vi "Write perform dynamic reads.vi"(8 "error in":errorcluster, 10 "perform dynamic reads":bool, 11 "DecideProjectFeatures in":refnum<class "TagBusProcessingPluginFeatureDecider.lvclass">) -> (0 "error out":errorcluster, 3 "DecideProjectFeatures out":refnum<class "TagBusProcessingPluginFeatureDecider.lvclass">)   [LabVIEW 2013, in "TagBusProcessingPluginFeatureDecider.lvclass"]
uses:
  TagBusProcessingPluginFeatureDecider.lvclass
  TagBusProcessingPluginFeatureDecider.lvclass/TagBusProcessingPluginFeatureDecider.ctl
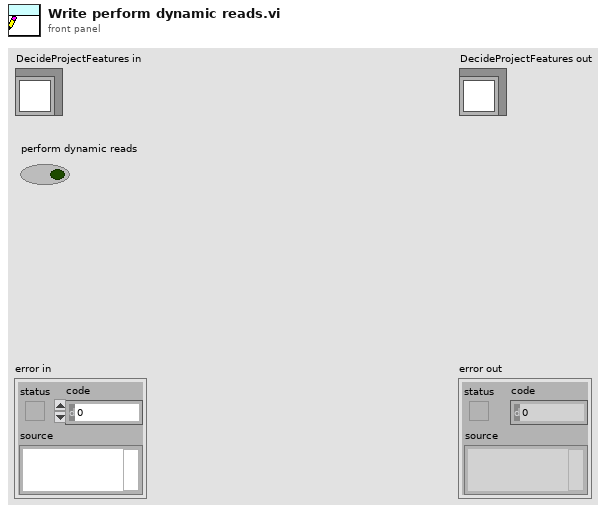
[diagram p1: front panel]
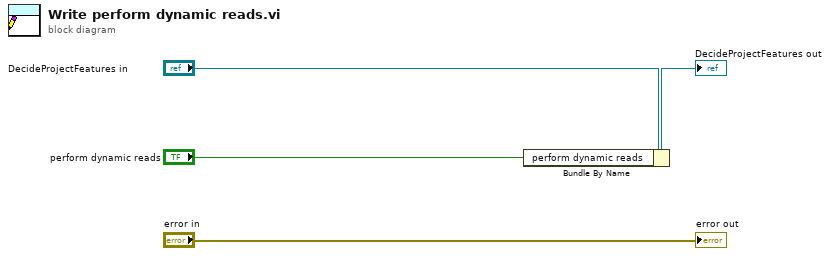
[diagram p0: block diagram]
diagram:
  n1 = Bundle By Name(cluster="DecideProjectFeatures in", "perform dynamic reads"="perform dynamic reads") -> (→"DecideProjectFeatures out":refnum<class "TagBusProcessingPluginFeatureDecider.lvclass">)
  "error out" <- "error in"
